vi "EV3Testing.vi"() -> ()   [LabVIEW 2019]
uses:
  <userlib>/MicroPython/VIs/uPythonX/uPythonX.xctl
panel:
  in  "Simple Beep":T1(xcontrol)={"Port"="169.254.244.73", "All Code"="#!/usr/bin/env pybricks-micropython\n\nfrom pybricks import ev3brick as brick\nfrom pybricks.ev3devices import (Motor, TouchSensor, ColorSensor,\n                                 InfraredSensor, UltrasonicSensor, GyroSensor)\nfrom pybricks.parameters import (Port, Stop, Direction, Button, Color,\n                                 SoundFile, ImageFile, Align)\nfrom pybricks.tools import print, wait, StopWatch\nfrom pybricks.robotics import DriveBase\n\n# Write your program here\nbrick.sound.beep()"}
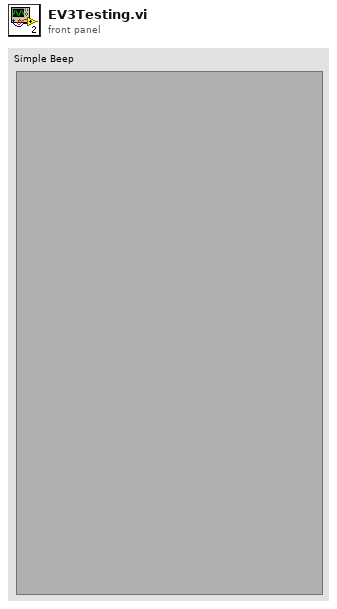
[diagram p1: front panel]
types:
  T1 = cluster{"Port":refnum<visa-resource-name>, "All Code":string}
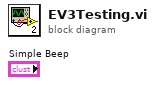
[diagram p0: block diagram]
diagram:
